vi "Stop Core.vi"(10 "final error code":i32, 11 "Base UI Actor in":refnum<class "Base UI Actor.lvclass">) -> (3 "Base UI Actor out":refnum<class "Base UI Actor.lvclass">)   [LabVIEW 2016, in "Assert API Components.lvlib" / "Base UI Actor.lvlib" / "Base UI Actor.lvclass"]
doc: "(<B>Filename</B>: Actor Framework.lvlib:Actor.lvclass:Stop Core.vi)\n\nDefines what the actor does before it stops. Use the <B>final error code</B> input to determine whether the actor shut down in response to an error.\n\nBy default, this method does nothing. A descendant class may override it to define behavior, such as shutting down any processes the actor initiated in its override of the Actor Core method."
uses:
  Base UI Actor.lvclass
  Base UI Actor.lvclass/Base UI Actor.ctl
  <vilib>/ActorFramework/Actor/Actor.lvclass
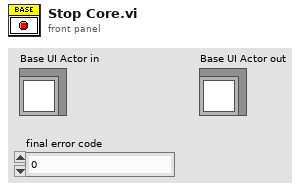
[diagram p1: front panel]
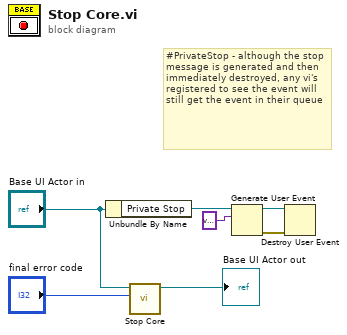
[diagram p0: block diagram]
diagram:
  # "#PrivateStop - although the stop message is generated and then immediately destroyed, any vi's registered to see the event will still get the event in their queue"
  n1 = Unbundle By Name("Base UI Actor in") -> ("Private Stop"=w4:refnum<user-event>)
  n2 = call-parent "Stop Core.vi"("final error code"="final error code", "Actor in"="Base UI Actor in") -> ("Actor out"=→"Base UI Actor out":refnum<class "Base UI Actor.lvclass">)  [unwired: 9 in]
  n3 = Generate User Event(user event=w4, event data cluster=variant ("event data")) -> (user event out=w2:refnum<user-event>, error out=w1:errorcluster)  [unwired: 2 in]
  n4 = Destroy User Event(user event=w2, error in=w1) -> ()  [unwired: 1 out]
